vi "ObtainBroadcastEvents.vi"(8 "ErrorArray In":errorcluster[](array[cluster])) -> (0 "ErrorArray Out":errorcluster[](array[cluster]), 3 "NISTBusBroadcast":T1)   [LabVIEW 2014, in "Bus.lvlib"]
uses:
  Bus.lvlib
  Typedefs/clBroadcastEvents.ctl
  Typedefs/clUserEventType.ctl
  <userlib>/NIST/NISTErrorLib/NISTErrorLib.lvlib
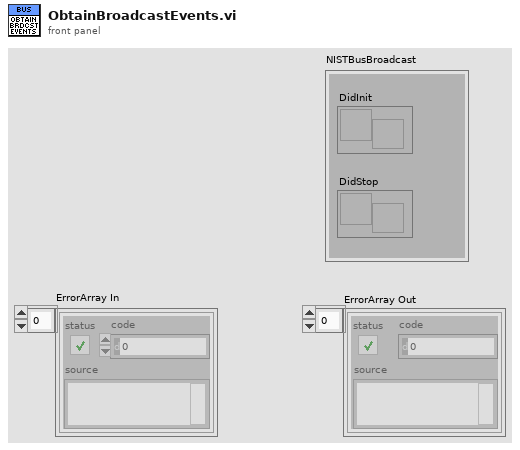
[diagram p1: front panel]
types:
  T1 = typedef "Bus.lvlib/clBroadcastEvents.ctl" = cluster{"DidInit":refnum<user-event>, "DidStop":refnum<user-event>}
  T2 = typedef "NISTBus.lvlib/clBroadcastEvents.ctl" = cluster{"DidInit":refnum<user-event>, "DidStop":refnum<user-event>}
  T3 = typedef "Bus.lvlib/clUserEventType.ctl" = cluster{"BusNumber":i8, "Data":variant}
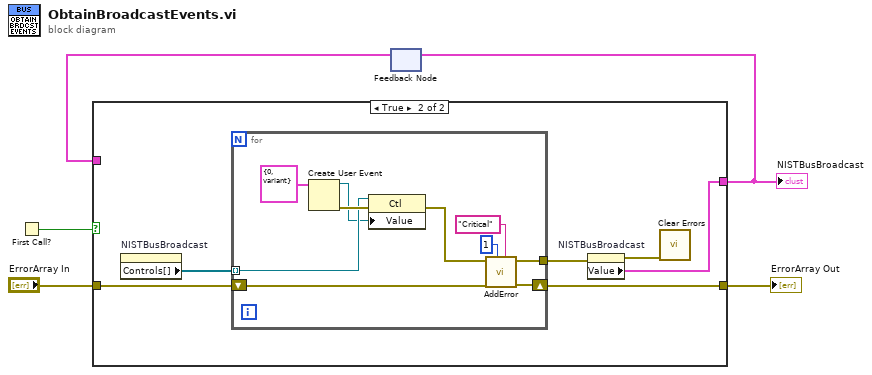
[diagram p0: block diagram]
diagram:
  n1 = First Call?() -> (First Call?: T/F=w5:bool)
  n2 = feedback #1() -> (w1:T2)  [unwired: 1 in]
  n3 = case shown="True" w5 {
    tunnel: "ErrorArray In" -> [w6 w12]
    tunnel: [w6 w11] -> w3
    tunnel: [w7 w8] -> w2
    tunnel: w1 -> [w7 _]
    frame False {
    }
    frame True {
      n4 = property on="NISTBusBroadcast" class="Clust (strict)"() -> ("Controls[]"=w13:refnum<vi>[])  [unwired: 2 in, 2 out]
      n5 = for {
        tunnel: w13 -> [w18] mode=indexing
        shift-right: [w15] -> w11
        shift-left: w12 -> [w16]
        tunnel: [w14] -> w10
        n6 = Create User Event(user event datatype=T3 {"BusNumber"=0, "Data"=variant} ("clEventType")) -> (user event=w17:refnum<user-event>, error out=w20:errorcluster)  [unwired: 1 in]
        n7 = property class="Ctl"(reference=w18, error in=w20, "Value"=w17) -> (error out=w19:errorcluster)  [unwired: 1 out]
        n8 = call <userlib>:"AddError.vi"("Severity"="Critical" ("String"), "Priority"=u8 1, "ErrorArray"=w16, "error in (no error)"=w19) -> ("ErrorArray"=w15:errorcluster[], "error out"=w14:errorcluster)  [unwired: 6 in]
      }
      n9 = property on="NISTBusBroadcast" class="Clust (strict)"(error in=w10) -> (error out=w9:errorcluster, "Value"=w8:T2)  [unwired: 1 in, 1 out]
      n10 = call <vilib>:"Clear Errors.vi"("error in (no error)"=w9) -> ()  [unwired: 5 in, 2 out]
    }
  }
  "NISTBusBroadcast" <- w2
  "ErrorArray Out" <- w3
  n11 = feedback-in #1(w2) -> ()
